vi "CCM-Read Connection Table.vi"(0 "Path In":path, 2 "Type":T2, 7 "IOChannels":string[](array[string]), 11 "error in (no error)":errorcluster) -> (4 "Path Out":path, 6 "Endpoints (by channel)":string[](array[string]), 10 "Table":T1[](array[typedef]), 15 "error out":errorcluster)   [LabVIEW 2020]
uses:
  Type Defs/CM-IO Type.ctl
  Type Defs/CM-Connection.ctl
  <vilib>/Utility/config.llb/Read Key (String).vi
  <vilib>/Utility/config.llb/NI_LVConfig.lvlib
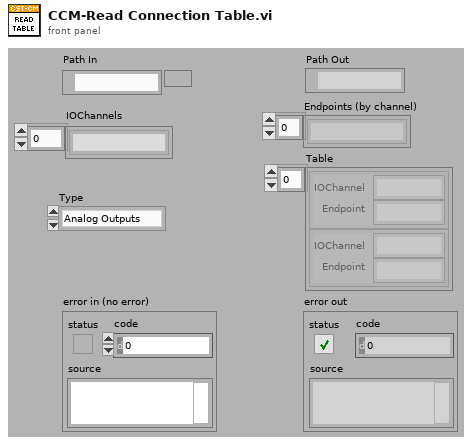
[diagram p1: front panel]
types:
  T1 = typedef "CM-Connection.ctl" = cluster{"IOChannel":string, "Endpoint":string}
  T2 = typedef "CM-IO Type.ctl" = enum16{"Analog Outputs", "Analog Inputs", "Digital Outputs", "Digital Inputs"}
  T3 = typedef "NI_LVConfig.lvlib/Config Data RefNum.ctl" = refnum<k1>
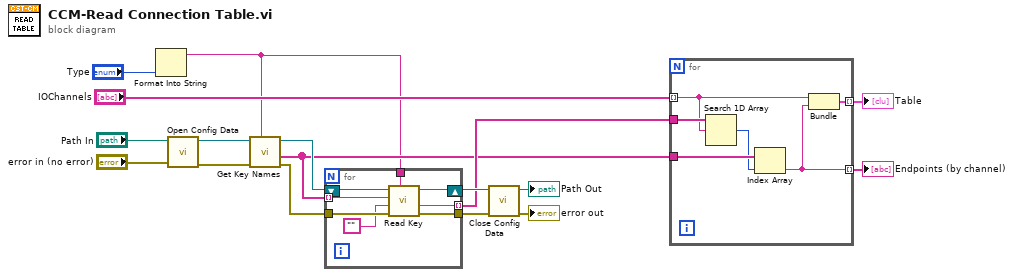
[diagram p0: block diagram]
diagram:
  n1 = Format Into String("Type") -> (resulting string=w1:string)  [unwired: 3 in, 1 out]
  n2 = call <vilib>:"Open Config Data.vi"("error in (no error)"="error in (no error)", "configuration file path"="Path In") -> ("error out"=w12:errorcluster, "refnum"=w13:T3)  [unwired: 7 in, 1 out]
  n3 = call <vilib>:"Get Key Names.vi"("section"=w1, "error in (no error)"=w12, "refnum"=w13) -> ("error out"=w10:errorcluster, "key names"=w4:string[], "refnum out"=w11:T3)  [unwired: 5 in, 1 out]
  n4 = for {
    tunnel: w10 -> [w23]
    tunnel: w4 -> [w24] mode=indexing
    tunnel: w1 -> [w21]
    tunnel: [w20] -> w6 mode=indexing
    tunnel: [w18] -> w8
    shift-right: [w19] -> w9
    shift-left: w11 -> [w25]
    n5 = call-poly <vilib>:"Read Key.vi"("section"=w21, "error in (no error)"=w23, "default value"="", "key"=w24, "refnum"=w25) -> ("error out"=w18:errorcluster, "value"=w20:string, "refnum out"=w19:T3)  [unwired: 3 in, 1 out]
  }
  n6 = call <vilib>:"Close Config Data.vi"("error in (no error)"=w8, "refnum"=w9) -> ("error out"=→"error out":errorcluster, "file path"=→"Path Out":path)  [unwired: 8 in]
  n7 = for {
    tunnel: "IOChannels" -> [w28] mode=indexing
    tunnel: w6 -> [w31]
    tunnel: w4 -> [w30]
    tunnel: [w27] -> w7 mode=indexing
    tunnel: [w26] -> w3 mode=indexing
    n8 = Search 1D Array(1D array=w31, element=w28) -> (index of element=w29:i32)  [unwired: 1 in]
    n9 = Index Array(array=w30, index=w29) -> (element=w26:string)
    n10 = Bundle("String"=w28, "String"=w26) -> (w27:cluster{"String":string, "String":string})  [unwired: 1 in]
  }
  "Table" <- w7
  "Endpoints (by channel)" <- w3
